vi "_DRIVER_SHARED_INI_VariantToLegibleString.vi"(6 "Format Options":T2, 7 "Preferred Units":T1(array[ring])=[enum."°", enum."m", enum."m²", enum."L", enum."m/s", enum."m/s²", enum."°/s", enum."°/s²", enum."kg", enum."s", enum."Hz", enum."°C", enum."bar", enum."N", enum."kg/m³", enum."N·m", enum."kg·m²", enum."V", enum."A", enum."W", enum."ohm", enum."µF", enum."mH", enum."kW·h", enum."lx", enum."C", enum."eV", enum."Gy", enum."lm", enum."S", enum."T"], 8 "error in (no error)":errorcluster, 11 "Variant":variant) -> (0 "error out":errorcluster, 1 "Var_Value":string, 2 "Var_name":string, 3 "String":string)   [LabVIEW 2020]
doc: "Converts almost anything in the form of a variant into a single line, legible string. Use <b>Format Options</b> to configure the output options. <b>Preferred Units</b> is only used when converting numerics with units. Select the preferred units from the list. If a compatible unit is not found, the base SI units are used."
uses:
  <vilib>/Utility/Data Type/Type Definitions/Data Type.ctl
  <vilib>/Utility/Data Type/NI_Data Type.lvlib
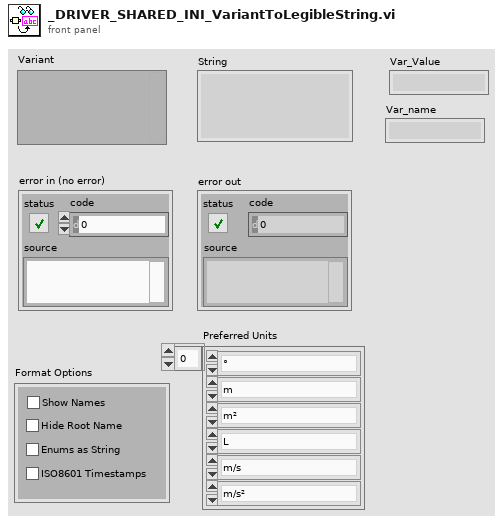
[diagram p1: front panel]
types:
  T1 = enum16{"---- Angle ----", "°", "'", "\"", "rad", "sr", "---- Length ----", "km", "m", "cm", "mm", "µm", "mi", "yd", "ft", "in", "---- Area ----", "ha", "m²", "cm²", "mm²", "µm²", "acre", "yd²", "ft²", "in²", "----Volume ----", "L", "m³", "cm³", "mm³", "gal", "pint", "ft³", "in³", "---- Velocity ----", "km/h", "m/s", "mm/s", "mi/h", "ft/min", "ft/s", "in/s", "---- Accelleration ----", "m/s²", "mm/s²", "ft/s²", "in/s²", "---- Angular Velocity ----", "°/s", "rad/s", "---- Angular Acceleration ----", "°/s²", "rad/s²", "---- Mass ----", "t", "kg", "g", "mg", "µg", "ton", "stone", "lb", "oz", "---- Time ----", "y", "d", "h", "min", "s", "ms", "µs", "ns", "---- Frequency ----", "GHz", "MHz", "kHz", "Hz", "---- Temperature ----", "K", "°C", "°F", "----Pressure ----", "atm", "bar", "mbar", "kPa", "Pa", "mm·Hg", "psi", "---- Force ----", "N", "lbf", "---- Density ----", "g/L", "g/100mL", "mg/L", "kg/m³", "g/cm³", "slug/ft³", "lb/ft³", "---- Torque ----", "N·m", "cN·m", "mN·m", "lb·ft", "oz·in", "---- Inertia ----", "kg·m²", "g·cm²", "lb·ft·s²", "---- Voltage ----", "kV", "V", "mV", "µV", "---- Current ----", "A", "mA", "µA", "---- Power ----", "MW", "kW", "W", "mW", "hp", "---- Resistance ----", "Mohm", "kohm", "ohm", "---- Capacitance ----", "F", "mF", "µF", "nF", "pF", "---- Inductance ----", "H", "mH", "µH", "---- Energy ----", "kW·h", "kJ", "J", "cal", "Btu", "---- Illuminance ----", "lx", "fc", "---- Other ----", "C", "eV", "Gy", "lm", "S", "T"}[]
  T2 = cluster{"Show Names":bool, "Hide Root Name":bool, "Enums as String":bool, "ISO8601 Timestamps":bool}
  T3 = typedef "NI_Data Type.lvlib/Data Type.ctl" = enum8{"Invalid Type", "Void", "I8", "I16", "I32", "I64", "U8", "U16", "U32", "U64", "Single Float", "Double Float", "Extended Float", "Single Complex", "Double Complex", "Extended Complex", "Enum U8", "Enum U16", "Enum U32", "Enum U64", "Single Float With Unit", "Double Float With Unit", "Extended Float With Unit", "Single Complex with Unit", "Double Complex with Unit", "Extended Complex with Unit", "Boolean", "String", "Path", "Picture", "Tag", "Array", "Cluster", "Variant", "LV Variant", "Waveform", "Timestamp", "Digital Waveform", "Digital Data", "ExpressData", "Refnum", "External Data", "VI", "Poly VI", "LabVIEW Class Instance", "Fixed Point", "Set Collection", "Map Collection"}
  T4 = typedef "NI_Data Type.lvlib/Unit Info.ctl" = cluster{"Unit Type":T5, "Exponent":i16}
  T5 = typedef "NI_Data Type.lvlib/Unit Type.ctl" = enum16{"Radians", "Steradians", "Seconds", "Meters", "Kilograms", "Amperes", "Kelvins", "Moles", "Candelas", "InvalidUnit"}
  T6 = typedef "LVFixedPointRepBitsTypeDef.ctl" = cluster{"Signed":bool, "Word Length":u32, "Integer Word Length":i32}
  T7 = typedef "NI_Data Type.lvlib/Refnum Type.ctl" = enum16{"NotARefnum", "UnknownRefnum", "Generic", "Datalog", "ByteStream", "Device", "Occurence", "TCPNetConnection", "Auto", "Menu", "Imaq", "Hardware", "DataSocket", "Visa", "IVI", "UDPNetConnection", "Notifier", "Queue", "Irda", "EventReg", "DotNet", "UserEvent", "Callback", "UNUSED_EMPTY_POSITION", "BlueToothNetConnection", "LVObjApp", "LVObjVI", "LVObjUnknown", "GenericClass", "UserDefinedRefnumTag", "DataValue", "RT FIFO", "TDMS File", "PythonSessionRefnum"}
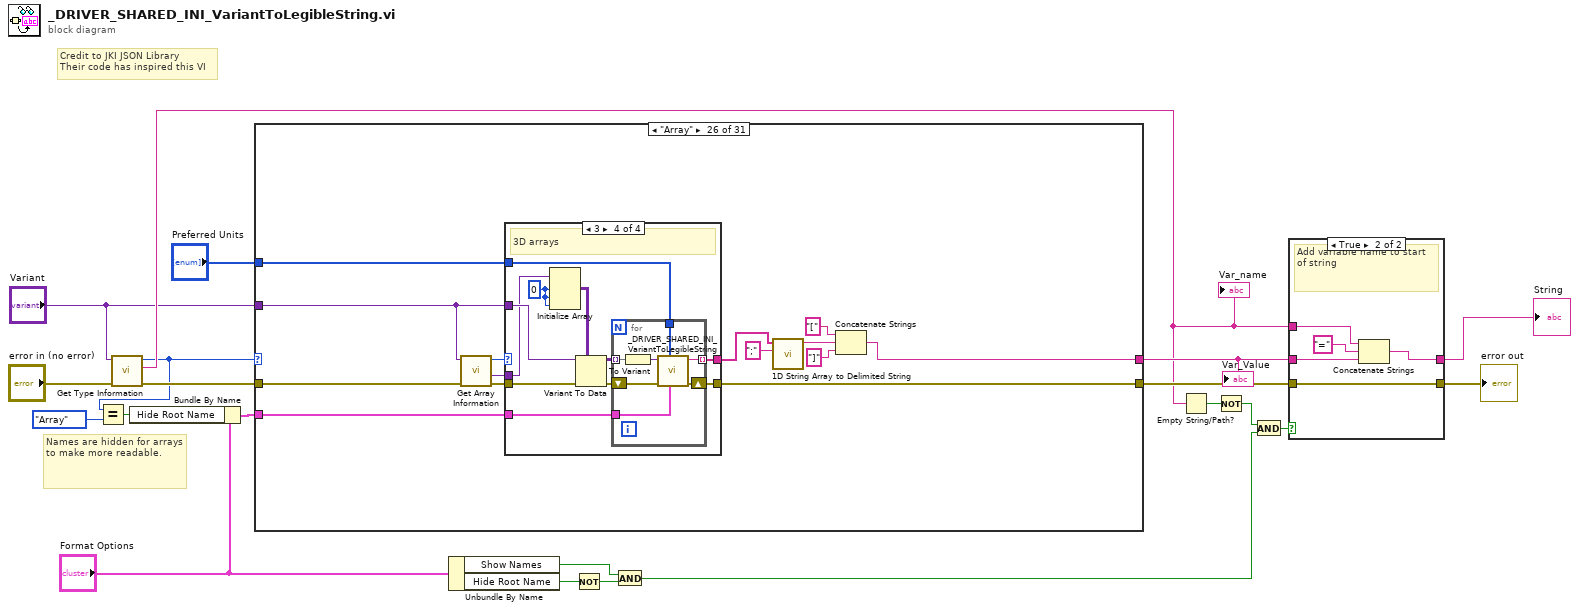
[diagram p0: block diagram]
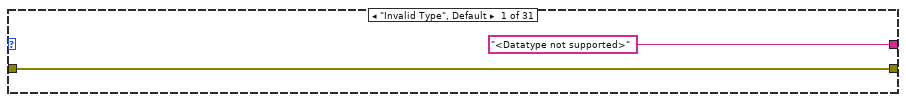
[diagram p3: hidden frame]
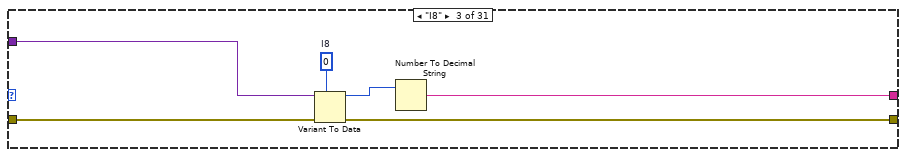
[diagram p5: hidden frame]
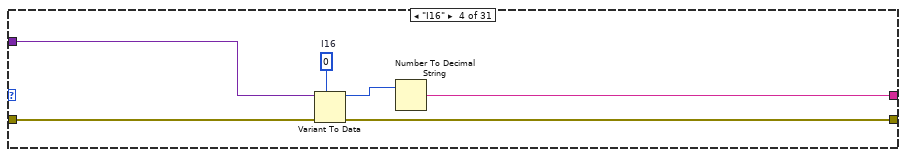
[diagram p6: hidden frame]
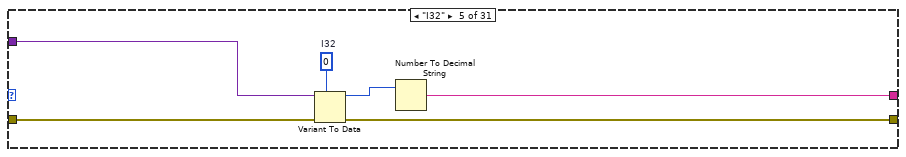
[diagram p7: hidden frame]
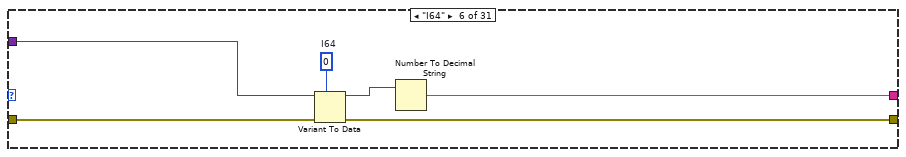
[diagram p8: hidden frame]
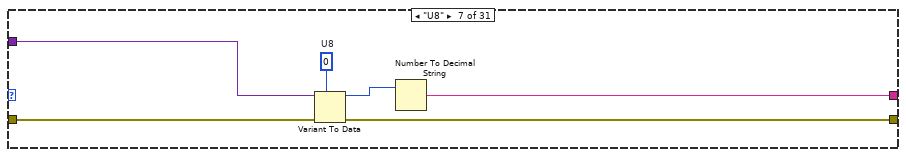
[diagram p9: hidden frame]
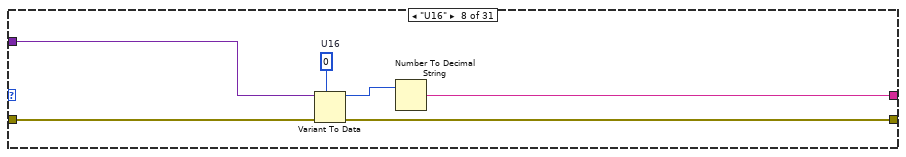
[diagram p10: hidden frame]
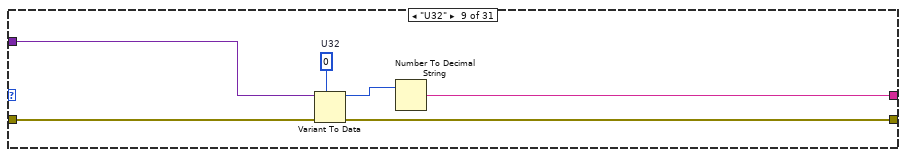
[diagram p11: hidden frame]
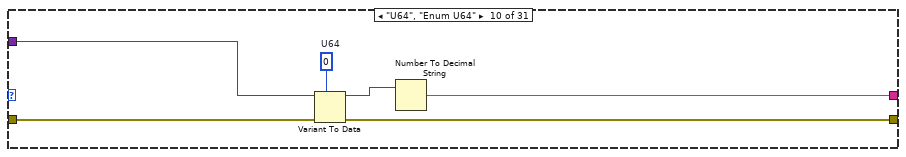
[diagram p12: hidden frame]
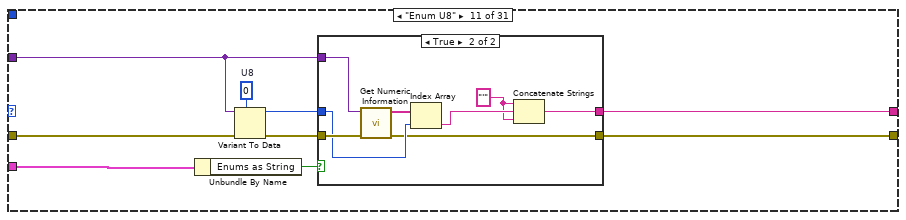
[diagram p13: hidden frame]
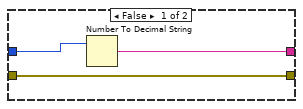
[diagram p14: hidden frame]
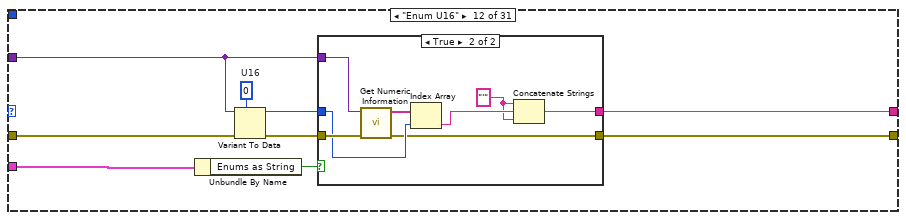
[diagram p15: hidden frame]
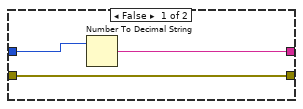
[diagram p16: hidden frame]
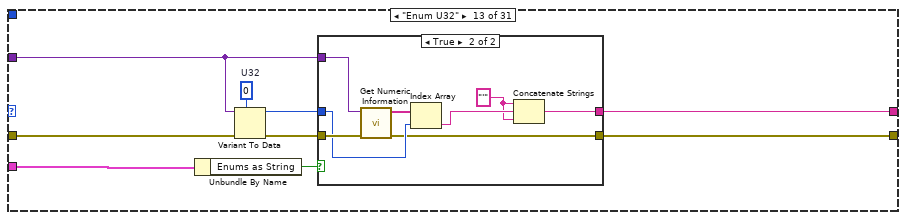
[diagram p17: hidden frame]
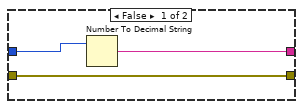
[diagram p18: hidden frame]
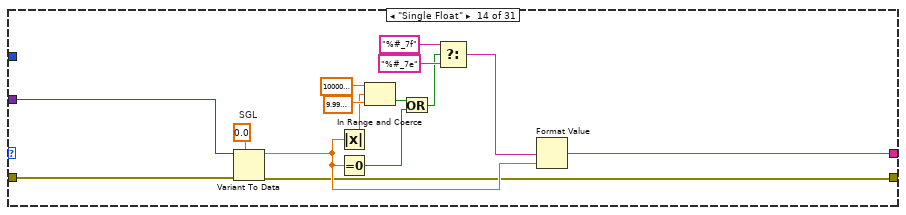
[diagram p19: hidden frame]
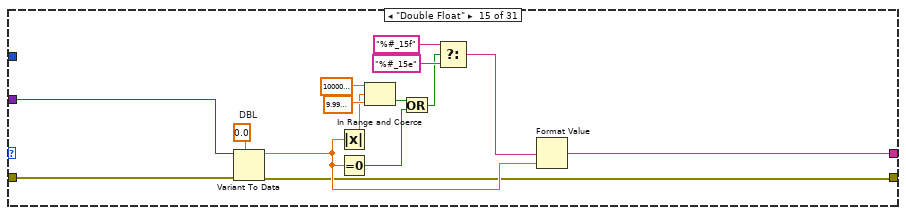
[diagram p20: hidden frame]
diagram:
  # "Names are hidden for arrays  to make more readable."
  # "Credit to JKI JSON Library\nTheir code has inspired this VI"
  n1 = call <vilib>:"Get Type Information.vi"("error in (no error)"="error in (no error)", "variant"="Variant") -> ("error out"=w20:errorcluster, "name"=w15:string, "type"=w5:T3)  [unwired: 5 in, 2 out]
  "Var_name" <- w15
  n2 = Equal?(x=w5, y=Data_Type."Array") -> (x = y?=w3:bool)
  n3 = Bundle By Name(cluster="Format Options", "Hide Root Name"=w3) -> (w6:T2)
  n4 = case shown="\"Array\"" w5 {
    selector: w5 -> [_ _ _ _ _ _ _ _ _ _ _ _ _ _ _ _ w190 _ _ _ _ _ _ _ _ _ _ _ _ _ _]
    tunnel: ["<Datatype not supported>" ("format string") _ w26 w32 w38 w44 w50 w56 w62 w68 w78 w98 w118 w134 w149 w164 w187 w960 w985 w1010 w1046 w1056 w1065 w1074 w1089 w1103 w1173 w1202 w1206 w1235 w1267] -> w16
    tunnel: [w23 w24 w25 w31 w37 w43 w49 w55 w61 w67 w75 w95 w115 w133 w148 w163 w191 w975 w1000 w1025 w1045 w1058 w1064 w1073 w1092 w1112 w1175 w1204 w1207 w1236 w1268] -> w18
    tunnel: w20 -> [w23 w24 w28 w34 w40 w46 w52 w58 w64 w70 w79 w99 w119 w138 w153 w168 w182 w978 w1003 w1028 w1043 w1059 w1069 w1078 w1093 w1113 w1174 w1203 w1213 w1234 w1272]
    tunnel: "Variant" -> [_ _ w27 w33 w39 w45 w51 w57 w63 w69 w76 w96 w116 w137 w152 w167 w180 w977 w1002 w1027 w1041 w1057 w1068 w1077 w1082 w1110 w1172 w1201 w1212 w1231 w1270]
    tunnel: w6 -> [_ _ _ _ _ _ _ _ _ _ w74 w94 w114 _ _ _ _ _ _ _ _ _ _ _ w1086 w1101 w1171 w1191 w1210 _ _]
    tunnel: "Preferred Units" -> [_ _ _ _ _ _ _ _ _ _ _ _ _ _ _ _ w183 _ _ _ _ _ _ _ w1079 w1100 w1170 w1190 _ _ _]
    frame "Invalid Type", Default {
    }
    frame "Void" {
    }
    frame "I8" {
      w29 = i8 0  # I8
      n5 = Variant To Data(error in=w28, type=w29, Variant=w27) -> (data=w30:i8, error out=w25:errorcluster)
      n6 = Number To Decimal String(number=w30) -> (decimal integer string=w26:string)  [unwired: 1 in]
    }
    frame "I16" {
      w35 = i16 0  # I16
      n7 = Variant To Data(error in=w34, type=w35, Variant=w33) -> (data=w36:i16, error out=w31:errorcluster)
      n8 = Number To Decimal String(number=w36) -> (decimal integer string=w32:string)  [unwired: 1 in]
    }
    frame "I32" {
      w41 = 0  # I32
      n9 = Variant To Data(error in=w40, type=w41, Variant=w39) -> (data=w42:i32, error out=w37:errorcluster)
      n10 = Number To Decimal String(number=w42) -> (decimal integer string=w38:string)  [unwired: 1 in]
    }
    frame "I64" {
      w47 = i64 0  # I64
      n11 = Variant To Data(error in=w46, type=w47, Variant=w45) -> (data=w48:i64, error out=w43:errorcluster)
      n12 = Number To Decimal String(number=w48) -> (decimal integer string=w44:string)  [unwired: 1 in]
    }
    frame "U8" {
      w53 = u8 0  # U8
      n13 = Variant To Data(error in=w52, type=w53, Variant=w51) -> (data=w54:u8, error out=w49:errorcluster)
      n14 = Number To Decimal String(number=w54) -> (decimal integer string=w50:string)  [unwired: 1 in]
    }
    frame "U16" {
      w59 = u16 0  # U16
      n15 = Variant To Data(error in=w58, type=w59, Variant=w57) -> (data=w60:u16, error out=w55:errorcluster)
      n16 = Number To Decimal String(number=w60) -> (decimal integer string=w56:string)  [unwired: 1 in]
    }
    frame "U32" {
      w65 = u32 0  # U32
      n17 = Variant To Data(error in=w64, type=w65, Variant=w63) -> (data=w66:u32, error out=w61:errorcluster)
      n18 = Number To Decimal String(number=w66) -> (decimal integer string=w62:string)  [unwired: 1 in]
    }
    frame "U64", "Enum U64" {
      w71 = u64 0  # U64
      n19 = Variant To Data(error in=w70, type=w71, Variant=w69) -> (data=w72:u64, error out=w67:errorcluster)
      n20 = Number To Decimal String(number=w72) -> (decimal integer string=w68:string)  [unwired: 1 in]
    }
    frame "Enum U8" {
      w80 = u8 0  # U8
      n21 = Unbundle By Name(w74) -> ("Enums as String"=w73:bool)
      n22 = Variant To Data(error in=w79, type=w80, Variant=w76) -> (data=w81:u8, error out=w77:errorcluster)
      n23 = case shown="True" w73 {
        tunnel: w81 -> [w84 w89]
        tunnel: [w83 w86] -> w78
        tunnel: w77 -> [w82 w92]
        tunnel: w76 -> [_ w91]
        tunnel: [w82 w88] -> w75
        frame False {
          n24 = Number To Decimal String(number=w84) -> (decimal integer string=w83:string)  [unwired: 1 in]
        }
        frame True {
          w85 = "'" ("string")
          n25 = call <vilib>:"Get Numeric Information.vi"("error in (no error)"=w92, "variant"=w91) -> ("error out"=w88:errorcluster, "enum names"=w90:string[])  [unwired: 6 in, 2 out]
          n26 = Index Array(array=w90, index=w89) -> (element=w87:string)
          n27 = Concatenate Strings(w85, w87, w85) -> (w86:string)
        }
      }
    }
    frame "Enum U16" {
      w100 = u16 0  # U16
      n28 = Unbundle By Name(w94) -> ("Enums as String"=w93:bool)
      n29 = Variant To Data(error in=w99, type=w100, Variant=w96) -> (data=w101:u16, error out=w97:errorcluster)
      n30 = case shown="True" w93 {
        tunnel: w101 -> [w104 w109]
        tunnel: [w103 w106] -> w98
        tunnel: w97 -> [w102 w112]
        tunnel: w96 -> [_ w111]
        tunnel: [w102 w108] -> w95
        frame False {
          n31 = Number To Decimal String(number=w104) -> (decimal integer string=w103:string)  [unwired: 1 in]
        }
        frame True {
          w105 = "'" ("string")
          n32 = call <vilib>:"Get Numeric Information.vi"("error in (no error)"=w112, "variant"=w111) -> ("error out"=w108:errorcluster, "enum names"=w110:string[])  [unwired: 6 in, 2 out]
          n33 = Index Array(array=w110, index=w109) -> (element=w107:string)
          n34 = Concatenate Strings(w105, w107, w105) -> (w106:string)
        }
      }
    }
    frame "Enum U32" {
      w120 = u32 0  # U32
      n35 = Unbundle By Name(w114) -> ("Enums as String"=w113:bool)
      n36 = Variant To Data(error in=w119, type=w120, Variant=w116) -> (data=w121:u32, error out=w117:errorcluster)
      n37 = case shown="True" w113 {
        tunnel: w121 -> [w124 w129]
        tunnel: [w123 w126] -> w118
        tunnel: w117 -> [w122 w132]
        tunnel: w116 -> [_ w131]
        tunnel: [w122 w128] -> w115
        frame False {
          n38 = Number To Decimal String(number=w124) -> (decimal integer string=w123:string)  [unwired: 1 in]
        }
        frame True {
          w125 = "'" ("string")
          n39 = call <vilib>:"Get Numeric Information.vi"("error in (no error)"=w132, "variant"=w131) -> ("error out"=w128:errorcluster, "enum names"=w130:string[])  [unwired: 6 in, 2 out]
          n40 = Index Array(array=w130, index=w129) -> (element=w127:string)
          n41 = Concatenate Strings(w125, w127, w125) -> (w126:string)
        }
      }
    }
    frame "Single Float" {
      w147 = sgl 0.0  # SGL
      n42 = Variant To Data(error in=w138, type=w147, Variant=w137) -> (data=w136:sgl, error out=w133:errorcluster)
      n43 = Absolute Value(x=w136) -> (abs(x)=w143:sgl)
      n44 = Equal To 0?(x=w136) -> (x = 0?=w142:bool)
      n45 = In Range and Coerce(upper limit=1000000.0, x=w143, lower limit=9.999999747378752e-05 ("upper limit")) -> (In Range?=w141:bool)  [unwired: 1 out]
      n46 = Or(x=w141, y=w142) -> (x .or. y?=w140:bool)
      n47 = Select(t="%#_7f" ("format string"), s=w140, f="%#_7e" ("format string")) -> (s? t:f=w135:string)
      n48 = Format Value(format string=w135, value (0)=w136) -> (output string=w134:string)  [unwired: 1 in]
    }
    frame "Double Float" {
      w162 = 0.0  # DBL
      n49 = Variant To Data(error in=w153, type=w162, Variant=w152) -> (data=w151:dbl, error out=w148:errorcluster)
      n50 = Absolute Value(x=w151) -> (abs(x)=w158:dbl)
      n51 = Equal To 0?(x=w151) -> (x = 0?=w157:bool)
      n52 = In Range and Coerce(upper limit=1000000.0, x=w158, lower limit=9.999999747378752e-05 ("upper limit")) -> (In Range?=w156:bool)  [unwired: 1 out]
      n53 = Or(x=w156, y=w157) -> (x .or. y?=w155:bool)
      n54 = Select(t="%#_15f" ("format string"), s=w155, f="%#_15e" ("format string")) -> (s? t:f=w150:string)
      n55 = Format Value(format string=w150, value (0)=w151) -> (output string=w149:string)  [unwired: 1 in]
    }
    frame "Extended Float" {
      w177 = ext 0.0  # EXT
      n56 = Variant To Data(error in=w168, type=w177, Variant=w167) -> (data=w166:ext, error out=w163:errorcluster)
      n57 = Absolute Value(x=w166) -> (abs(x)=w173:ext)
      n58 = Equal To 0?(x=w166) -> (x = 0?=w172:bool)
      n59 = In Range and Coerce(upper limit=1000000.0, x=w173, lower limit=9.999999747378752e-05 ("upper limit")) -> (In Range?=w171:bool)  [unwired: 1 out]
      n60 = Or(x=w171, y=w172) -> (x .or. y?=w170:bool)
      n61 = Select(t="%#_18f" ("format string"), s=w170, f="%#_18e" ("format string")) -> (s? t:f=w165:string)
      n62 = Format Value(format string=w165, value (0)=w166) -> (output string=w164:string)  [unwired: 1 in]
    }
    frame "Single Float With Unit".."Extended Float With Unit" {
      # "Add any new units into this case and update the enum. Copy an existing case and rename with units of choice. The Enum label will become the unit text."
      n63 = for {
        tunnel: w183 -> [w194] mode=indexing
        tunnel: w180 -> [w195]
        tunnel: [w194] -> w181
        tunnel: [w193] -> w179
        tunnel: [w192] -> w178
        stop <- w193 continue-if-true
        # "Search for unit match"
        n64 = case shown="\"mm/s²\"" w194 {
          tunnel: w195 -> [_ w202 w207 w212 w217 w222 w227 w232 w237 w242 w247 w252 w257 w262 w267 w272 w277 w282 w287 w292 w297 w302 w307 w312 w317 w322 w327 w332 w337 w342 w347 w352 w357 w362 w367 w372 w377 w382 w387 w392 w397 w402 w407 w412 w417 w422 w427 w432 w437 w442 w447 w452 w457 w462 w467 w472 w477 w482 w487 w492 w497 w502 w507 w512 w517 w522 w527 w532 w537 w542 w547 w552 w557 w562 w567 w572 w577 w582 w587 w592 w597 w602 w607 w612 w617 w622 w627 w632 w637 w642 w647 w652 w657 w662 w667 w672 w677 w682 w687 w692 w697 w702 w707 w712 w717 w722 w727 w732 w737 w742 w747 w752 w757 w762 w767 w772 w777 w782 w787 w792 w797 w802 w807 w812 w817 w822 w827 w832 w837 w842 w847]
          tunnel: [errorcluster {"status"=TRUE, "code"=0, "source"=""} ("error out") w199 w204 w209 w214 w219 w224 w229 w234 w239 w244 w249 w254 w259 w264 w269 w274 w279 w284 w289 w294 w299 w304 w309 w314 w319 w324 w329 w334 w339 w344 w349 w354 w359 w364 w369 w374 w379 w384 w389 w394 w399 w404 w409 w414 w419 w424 w429 w434 w439 w444 w449 w454 w459 w464 w469 w474 w479 w484 w489 w494 w499 w504 w509 w514 w519 w524 w529 w534 w539 w544 w549 w554 w559 w564 w569 w574 w579 w584 w589 w594 w599 w604 w609 w614 w619 w624 w629 w634 w639 w644 w649 w654 w659 w664 w669 w674 w679 w684 w689 w694 w699 w704 w709 w714 w719 w724 w729 w734 w739 w744 w749 w754 w759 w764 w769 w774 w779 w784 w789 w794 w799 w804 w809 w814 w819 w824 w829 w834 w839 w844] -> w193
          tunnel: [ext 0.0 w198 w203 w208 w213 w218 w223 w228 w233 w238 w243 w248 w253 w258 w263 w268 w273 w278 w283 w288 w293 w298 w303 w308 w313 w318 w323 w328 w333 w338 w343 w348 w353 w358 w363 w368 w373 w378 w383 w388 w393 w398 w403 w408 w413 w418 w423 w428 w433 w438 w443 w448 w453 w458 w463 w468 w473 w478 w483 w488 w493 w498 w503 w508 w513 w518 w523 w528 w533 w538 w543 w548 w553 w558 w563 w568 w573 w578 w583 w588 w593 w598 w603 w608 w613 w618 w623 w628 w633 w638 w643 w648 w653 w658 w663 w668 w673 w678 w683 w688 w693 w698 w703 w708 w713 w718 w723 w728 w733 w738 w743 w748 w753 w758 w763 w768 w773 w778 w783 w788 w793 w798 w803 w808 w813 w818 w823 w828 w833 w838 w843] -> w192
          frame Default {
          }
          frame "°" {
            w201 = ext[unit] 0.0  # deg
            n65 = Variant To Data(type=w201, Variant=w202) -> (data=w200:ext[unit], error out=w199:errorcluster)  [unwired: 1 in]
            n66 = node(w200) -> (w198:ext)
          }
          frame "'" {
            w206 = ext[unit] 0.0  # '
            n67 = Variant To Data(type=w206, Variant=w207) -> (data=w205:ext[unit], error out=w204:errorcluster)  [unwired: 1 in]
            n68 = node(w205) -> (w203:ext)
          }
          frame "\"" {
            w211 = ext[unit] 0.0  # "
            n69 = Variant To Data(type=w211, Variant=w212) -> (data=w210:ext[unit], error out=w209:errorcluster)  [unwired: 1 in]
            n70 = node(w210) -> (w208:ext)
          }
          frame "rad" {
            w216 = ext[unit] 0.0  # rad
            n71 = Variant To Data(type=w216, Variant=w217) -> (data=w215:ext[unit], error out=w214:errorcluster)  [unwired: 1 in]
            n72 = node(w215) -> (w213:ext)
          }
          frame "sr" {
            w221 = ext[unit] 0.0  # sr
            n73 = Variant To Data(type=w221, Variant=w222) -> (data=w220:ext[unit], error out=w219:errorcluster)  [unwired: 1 in]
            n74 = node(w220) -> (w218:ext)
          }
          frame "km" {
            w226 = ext[unit] 0.0  # km
            n75 = Variant To Data(type=w226, Variant=w227) -> (data=w225:ext[unit], error out=w224:errorcluster)  [unwired: 1 in]
            n76 = node(w225) -> (w223:ext)
          }
          frame "m" {
            w231 = ext[unit] 0.0  # m
            n77 = Variant To Data(type=w231, Variant=w232) -> (data=w230:ext[unit], error out=w229:errorcluster)  [unwired: 1 in]
            n78 = node(w230) -> (w228:ext)
          }
          frame "cm" {
            w236 = ext[unit] 0.0  # cm
            n79 = Variant To Data(type=w236, Variant=w237) -> (data=w235:ext[unit], error out=w234:errorcluster)  [unwired: 1 in]
            n80 = node(w235) -> (w233:ext)
          }
          frame "mm" {
            w241 = ext[unit] 0.0  # mm
            n81 = Variant To Data(type=w241, Variant=w242) -> (data=w240:ext[unit], error out=w239:errorcluster)  [unwired: 1 in]
            n82 = node(w240) -> (w238:ext)
          }
          frame "µm" {
            w246 = ext[unit] 0.0  # um
            n83 = Variant To Data(type=w246, Variant=w247) -> (data=w245:ext[unit], error out=w244:errorcluster)  [unwired: 1 in]
            n84 = node(w245) -> (w243:ext)
          }
          frame "mi" {
            w251 = ext[unit] 0.0  # mi
            n85 = Variant To Data(type=w251, Variant=w252) -> (data=w250:ext[unit], error out=w249:errorcluster)  [unwired: 1 in]
            n86 = node(w250) -> (w248:ext)
          }
          frame "yd" {
            w256 = ext[unit] 0.0  # yd
            n87 = Variant To Data(type=w256, Variant=w257) -> (data=w255:ext[unit], error out=w254:errorcluster)  [unwired: 1 in]
            n88 = node(w255) -> (w253:ext)
          }
          frame "ft" {
            w261 = ext[unit] 0.0  # ft
            n89 = Variant To Data(type=w261, Variant=w262) -> (data=w260:ext[unit], error out=w259:errorcluster)  [unwired: 1 in]
            n90 = node(w260) -> (w258:ext)
          }
          frame "in" {
            w266 = ext[unit] 0.0  # in
            n91 = Variant To Data(type=w266, Variant=w267) -> (data=w265:ext[unit], error out=w264:errorcluster)  [unwired: 1 in]
            n92 = node(w265) -> (w263:ext)
          }
          frame "ha" {
            w271 = ext[unit] 0.0  # ha
            n93 = Variant To Data(type=w271, Variant=w272) -> (data=w270:ext[unit], error out=w269:errorcluster)  [unwired: 1 in]
            n94 = node(w270) -> (w268:ext)
          }
          frame "m²" {
            w276 = ext[unit] 0.0  # m^2
            n95 = Variant To Data(type=w276, Variant=w277) -> (data=w275:ext[unit], error out=w274:errorcluster)  [unwired: 1 in]
            n96 = node(w275) -> (w273:ext)
          }
          frame "cm²" {
            w281 = ext[unit] 0.0  # cm^2
            n97 = Variant To Data(type=w281, Variant=w282) -> (data=w280:ext[unit], error out=w279:errorcluster)  [unwired: 1 in]
            n98 = node(w280) -> (w278:ext)
          }
          frame "mm²" {
            w286 = ext[unit] 0.0  # mm^2
            n99 = Variant To Data(type=w286, Variant=w287) -> (data=w285:ext[unit], error out=w284:errorcluster)  [unwired: 1 in]
            n100 = node(w285) -> (w283:ext)
          }
          frame "µm²" {
            w291 = ext[unit] 0.0  # um^2
            n101 = Variant To Data(type=w291, Variant=w292) -> (data=w290:ext[unit], error out=w289:errorcluster)  [unwired: 1 in]
            n102 = node(w290) -> (w288:ext)
          }
          frame "acre" {
            w296 = ext[unit] 0.0  # acre
            n103 = Variant To Data(type=w296, Variant=w297) -> (data=w295:ext[unit], error out=w294:errorcluster)  [unwired: 1 in]
            n104 = node(w295) -> (w293:ext)
          }
          frame "yd²" {
            w301 = ext[unit] 0.0  # yd^2
            n105 = Variant To Data(type=w301, Variant=w302) -> (data=w300:ext[unit], error out=w299:errorcluster)  [unwired: 1 in]
            n106 = node(w300) -> (w298:ext)
          }
          frame "ft²" {
            w306 = ext[unit] 0.0  # ft^2
            n107 = Variant To Data(type=w306, Variant=w307) -> (data=w305:ext[unit], error out=w304:errorcluster)  [unwired: 1 in]
            n108 = node(w305) -> (w303:ext)
          }
          frame "in²" {
            w311 = ext[unit] 0.0  # in^2
            n109 = Variant To Data(type=w311, Variant=w312) -> (data=w310:ext[unit], error out=w309:errorcluster)  [unwired: 1 in]
            n110 = node(w310) -> (w308:ext)
          }
          frame "L" {
            w316 = ext[unit] 0.0  # l
            n111 = Variant To Data(type=w316, Variant=w317) -> (data=w315:ext[unit], error out=w314:errorcluster)  [unwired: 1 in]
            n112 = node(w315) -> (w313:ext)
          }
          frame "m³" {
            w321 = ext[unit] 0.0  # m^3
            n113 = Variant To Data(type=w321, Variant=w322) -> (data=w320:ext[unit], error out=w319:errorcluster)  [unwired: 1 in]
            n114 = node(w320) -> (w318:ext)
          }
          frame "cm³" {
            w326 = ext[unit] 0.0  # cm^3
            n115 = Variant To Data(type=w326, Variant=w327) -> (data=w325:ext[unit], error out=w324:errorcluster)  [unwired: 1 in]
            n116 = node(w325) -> (w323:ext)
          }
          frame "mm³" {
            w331 = ext[unit] 0.0  # mm^3
            n117 = Variant To Data(type=w331, Variant=w332) -> (data=w330:ext[unit], error out=w329:errorcluster)  [unwired: 1 in]
            n118 = node(w330) -> (w328:ext)
          }
          frame "gal" {
            w336 = ext[unit] 0.0  # gal
            n119 = Variant To Data(type=w336, Variant=w337) -> (data=w335:ext[unit], error out=w334:errorcluster)  [unwired: 1 in]
            n120 = node(w335) -> (w333:ext)
          }
          frame "pint" {
            w341 = ext[unit] 0.0  # pint
            n121 = Variant To Data(type=w341, Variant=w342) -> (data=w340:ext[unit], error out=w339:errorcluster)  [unwired: 1 in]
            n122 = node(w340) -> (w338:ext)
          }
          frame "ft³" {
            w346 = ext[unit] 0.0  # ft^3
            n123 = Variant To Data(type=w346, Variant=w347) -> (data=w345:ext[unit], error out=w344:errorcluster)  [unwired: 1 in]
            n124 = node(w345) -> (w343:ext)
          }
          frame "in³" {
            w351 = ext[unit] 0.0  # in^3
            n125 = Variant To Data(type=w351, Variant=w352) -> (data=w350:ext[unit], error out=w349:errorcluster)  [unwired: 1 in]
            n126 = node(w350) -> (w348:ext)
          }
          frame "km/h" {
            w356 = ext[unit] 0.0  # km/h
            n127 = Variant To Data(type=w356, Variant=w357) -> (data=w355:ext[unit], error out=w354:errorcluster)  [unwired: 1 in]
            n128 = node(w355) -> (w353:ext)
          }
          frame "m/s" {
            w361 = ext[unit] 0.0  # m/s
            n129 = Variant To Data(type=w361, Variant=w362) -> (data=w360:ext[unit], error out=w359:errorcluster)  [unwired: 1 in]
            n130 = node(w360) -> (w358:ext)
          }
          frame "mm/s" {
            w366 = ext[unit] 0.0  # mm/s
            n131 = Variant To Data(type=w366, Variant=w367) -> (data=w365:ext[unit], error out=w364:errorcluster)  [unwired: 1 in]
            n132 = node(w365) -> (w363:ext)
          }
          frame "mi/h" {
            w371 = ext[unit] 0.0  # mi/h
            n133 = Variant To Data(type=w371, Variant=w372) -> (data=w370:ext[unit], error out=w369:errorcluster)  [unwired: 1 in]
            n134 = node(w370) -> (w368:ext)
          }
          frame "ft/min" {
            w376 = ext[unit] 0.0  # ft/min
            n135 = Variant To Data(type=w376, Variant=w377) -> (data=w375:ext[unit], error out=w374:errorcluster)  [unwired: 1 in]
            n136 = node(w375) -> (w373:ext)
          }
          frame "ft/s" {
            w381 = ext[unit] 0.0  # ft/s
            n137 = Variant To Data(type=w381, Variant=w382) -> (data=w380:ext[unit], error out=w379:errorcluster)  [unwired: 1 in]
            n138 = node(w380) -> (w378:ext)
          }
          frame "in/s" {
            w386 = ext[unit] 0.0  # in/s
            n139 = Variant To Data(type=w386, Variant=w387) -> (data=w385:ext[unit], error out=w384:errorcluster)  [unwired: 1 in]
            n140 = node(w385) -> (w383:ext)
          }
          frame "m/s²" {
            w391 = ext[unit] 0.0  # m/s^2
            n141 = Variant To Data(type=w391, Variant=w392) -> (data=w390:ext[unit], error out=w389:errorcluster)  [unwired: 1 in]
            n142 = node(w390) -> (w388:ext)
          }
          frame "mm/s²" {
            w396 = ext[unit] 0.0  # mm/s^2
            n143 = Variant To Data(type=w396, Variant=w397) -> (data=w395:ext[unit], error out=w394:errorcluster)  [unwired: 1 in]
            n144 = node(w395) -> (w393:ext)
          }
          frame "ft/s²" {
            w401 = ext[unit] 0.0  # ft/s^2
            n145 = Variant To Data(type=w401, Variant=w402) -> (data=w400:ext[unit], error out=w399:errorcluster)  [unwired: 1 in]
            n146 = node(w400) -> (w398:ext)
          }
          frame "in/s²" {
            w406 = ext[unit] 0.0  # in/s^2
            n147 = Variant To Data(type=w406, Variant=w407) -> (data=w405:ext[unit], error out=w404:errorcluster)  [unwired: 1 in]
            n148 = node(w405) -> (w403:ext)
          }
          frame "°/s" {
            w411 = ext[unit] 0.0  # deg/s
            n149 = Variant To Data(type=w411, Variant=w412) -> (data=w410:ext[unit], error out=w409:errorcluster)  [unwired: 1 in]
            n150 = node(w410) -> (w408:ext)
          }
          frame "rad/s" {
            w416 = ext[unit] 0.0  # rad/s
            n151 = Variant To Data(type=w416, Variant=w417) -> (data=w415:ext[unit], error out=w414:errorcluster)  [unwired: 1 in]
            n152 = node(w415) -> (w413:ext)
          }
          frame "°/s²" {
            w421 = ext[unit] 0.0  # deg/s^2
            n153 = Variant To Data(type=w421, Variant=w422) -> (data=w420:ext[unit], error out=w419:errorcluster)  [unwired: 1 in]
            n154 = node(w420) -> (w418:ext)
          }
          frame "rad/s²" {
            w426 = ext[unit] 0.0  # rad/s^2
            n155 = Variant To Data(type=w426, Variant=w427) -> (data=w425:ext[unit], error out=w424:errorcluster)  [unwired: 1 in]
            n156 = node(w425) -> (w423:ext)
          }
          frame "t" {
            w431 = ext[unit] 0.0  # t
            n157 = Variant To Data(type=w431, Variant=w432) -> (data=w430:ext[unit], error out=w429:errorcluster)  [unwired: 1 in]
            n158 = node(w430) -> (w428:ext)
          }
          frame "kg" {
            w436 = ext[unit] 0.0  # kg
            n159 = Variant To Data(type=w436, Variant=w437) -> (data=w435:ext[unit], error out=w434:errorcluster)  [unwired: 1 in]
            n160 = node(w435) -> (w433:ext)
          }
          frame "g" {
            w441 = ext[unit] 0.0  # g
            n161 = Variant To Data(type=w441, Variant=w442) -> (data=w440:ext[unit], error out=w439:errorcluster)  [unwired: 1 in]
            n162 = node(w440) -> (w438:ext)
          }
          frame "mg" {
            w446 = ext[unit] 0.0  # mg
            n163 = Variant To Data(type=w446, Variant=w447) -> (data=w445:ext[unit], error out=w444:errorcluster)  [unwired: 1 in]
            n164 = node(w445) -> (w443:ext)
          }
          frame "µg" {
            w451 = ext[unit] 0.0  # ug
            n165 = Variant To Data(type=w451, Variant=w452) -> (data=w450:ext[unit], error out=w449:errorcluster)  [unwired: 1 in]
            n166 = node(w450) -> (w448:ext)
          }
          frame "ton" {
            w456 = ext[unit] 0.0  # ton
            n167 = Variant To Data(type=w456, Variant=w457) -> (data=w455:ext[unit], error out=w454:errorcluster)  [unwired: 1 in]
            n168 = node(w455) -> (w453:ext)
          }
          frame "stone" {
            w461 = ext[unit] 0.0  # stone
            n169 = Variant To Data(type=w461, Variant=w462) -> (data=w460:ext[unit], error out=w459:errorcluster)  [unwired: 1 in]
            n170 = node(w460) -> (w458:ext)
          }
          frame "lb" {
            w466 = ext[unit] 0.0  # lb
            n171 = Variant To Data(type=w466, Variant=w467) -> (data=w465:ext[unit], error out=w464:errorcluster)  [unwired: 1 in]
            n172 = node(w465) -> (w463:ext)
          }
          frame "oz" {
            w471 = ext[unit] 0.0  # oz
            n173 = Variant To Data(type=w471, Variant=w472) -> (data=w470:ext[unit], error out=w469:errorcluster)  [unwired: 1 in]
            n174 = node(w470) -> (w468:ext)
          }
          frame "y" {
            w476 = ext[unit] 0.0  # a
            n175 = Variant To Data(type=w476, Variant=w477) -> (data=w475:ext[unit], error out=w474:errorcluster)  [unwired: 1 in]
            n176 = node(w475) -> (w473:ext)
          }
          frame "d" {
            w481 = ext[unit] 0.0  # d
            n177 = Variant To Data(type=w481, Variant=w482) -> (data=w480:ext[unit], error out=w479:errorcluster)  [unwired: 1 in]
            n178 = node(w480) -> (w478:ext)
          }
          frame "h" {
            w486 = ext[unit] 0.0  # h
            n179 = Variant To Data(type=w486, Variant=w487) -> (data=w485:ext[unit], error out=w484:errorcluster)  [unwired: 1 in]
            n180 = node(w485) -> (w483:ext)
          }
          frame "min" {
            w491 = ext[unit] 0.0  # min
            n181 = Variant To Data(type=w491, Variant=w492) -> (data=w490:ext[unit], error out=w489:errorcluster)  [unwired: 1 in]
            n182 = node(w490) -> (w488:ext)
          }
          frame "s" {
            w496 = ext[unit] 0.0  # s
            n183 = Variant To Data(type=w496, Variant=w497) -> (data=w495:ext[unit], error out=w494:errorcluster)  [unwired: 1 in]
            n184 = node(w495) -> (w493:ext)
          }
          frame "ms" {
            w501 = ext[unit] 0.0  # ms
            n185 = Variant To Data(type=w501, Variant=w502) -> (data=w500:ext[unit], error out=w499:errorcluster)  [unwired: 1 in]
            n186 = node(w500) -> (w498:ext)
          }
          frame "µs" {
            w506 = ext[unit] 0.0  # us
            n187 = Variant To Data(type=w506, Variant=w507) -> (data=w505:ext[unit], error out=w504:errorcluster)  [unwired: 1 in]
            n188 = node(w505) -> (w503:ext)
          }
          frame "ns" {
            w511 = ext[unit] 0.0  # ns
            n189 = Variant To Data(type=w511, Variant=w512) -> (data=w510:ext[unit], error out=w509:errorcluster)  [unwired: 1 in]
            n190 = node(w510) -> (w508:ext)
          }
          frame "GHz" {
            w516 = ext[unit] 0.0  # GHz
            n191 = Variant To Data(type=w516, Variant=w517) -> (data=w515:ext[unit], error out=w514:errorcluster)  [unwired: 1 in]
            n192 = node(w515) -> (w513:ext)
          }
          frame "MHz" {
            w521 = ext[unit] 0.0  # MHz
            n193 = Variant To Data(type=w521, Variant=w522) -> (data=w520:ext[unit], error out=w519:errorcluster)  [unwired: 1 in]
            n194 = node(w520) -> (w518:ext)
          }
          frame "kHz" {
            w526 = ext[unit] 0.0  # kHz
            n195 = Variant To Data(type=w526, Variant=w527) -> (data=w525:ext[unit], error out=w524:errorcluster)  [unwired: 1 in]
            n196 = node(w525) -> (w523:ext)
          }
          frame "Hz" {
            w531 = ext[unit] 0.0  # Hz
            n197 = Variant To Data(type=w531, Variant=w532) -> (data=w530:ext[unit], error out=w529:errorcluster)  [unwired: 1 in]
            n198 = node(w530) -> (w528:ext)
          }
          frame "K" {
            w536 = ext[unit] 0.0  # K
            n199 = Variant To Data(type=w536, Variant=w537) -> (data=w535:ext[unit], error out=w534:errorcluster)  [unwired: 1 in]
            n200 = node(w535) -> (w533:ext)
          }
          frame "°C" {
            w541 = ext[unit] 273.15  # degC
            n201 = Variant To Data(type=w541, Variant=w542) -> (data=w540:ext[unit], error out=w539:errorcluster)  [unwired: 1 in]
            n202 = node(w540) -> (w538:ext)
          }
          frame "°F" {
            w546 = ext[unit] 255.3722222222222  # degF
            n203 = Variant To Data(type=w546, Variant=w547) -> (data=w545:ext[unit], error out=w544:errorcluster)  [unwired: 1 in]
            n204 = node(w545) -> (w543:ext)
          }
          frame "atm" {
            w551 = ext[unit] 0.0  # atm
            n205 = Variant To Data(type=w551, Variant=w552) -> (data=w550:ext[unit], error out=w549:errorcluster)  [unwired: 1 in]
            n206 = node(w550) -> (w548:ext)
          }
          frame "bar" {
            w556 = ext[unit] 0.0  # bar
            n207 = Variant To Data(type=w556, Variant=w557) -> (data=w555:ext[unit], error out=w554:errorcluster)  [unwired: 1 in]
            n208 = node(w555) -> (w553:ext)
          }
          frame "mbar" {
            w561 = ext[unit] 0.0  # mbar
            n209 = Variant To Data(type=w561, Variant=w562) -> (data=w560:ext[unit], error out=w559:errorcluster)  [unwired: 1 in]
            n210 = node(w560) -> (w558:ext)
          }
          frame "kPa" {
            w566 = ext[unit] 0.0  # kPa
            n211 = Variant To Data(type=w566, Variant=w567) -> (data=w565:ext[unit], error out=w564:errorcluster)  [unwired: 1 in]
            n212 = node(w565) -> (w563:ext)
          }
          frame "Pa" {
            w571 = ext[unit] 0.0  # Pa
            n213 = Variant To Data(type=w571, Variant=w572) -> (data=w570:ext[unit], error out=w569:errorcluster)  [unwired: 1 in]
            n214 = node(w570) -> (w568:ext)
          }
          frame "mm·Hg" {
            w576 = ext[unit] 0.0  # mm.Hg
            n215 = Variant To Data(type=w576, Variant=w577) -> (data=w575:ext[unit], error out=w574:errorcluster)  [unwired: 1 in]
            n216 = node(w575) -> (w573:ext)
          }
          frame "psi" {
            w581 = ext[unit] 0.0  # psi
            n217 = Variant To Data(type=w581, Variant=w582) -> (data=w580:ext[unit], error out=w579:errorcluster)  [unwired: 1 in]
            n218 = node(w580) -> (w578:ext)
          }
          frame "N" {
            w586 = ext[unit] 0.0  # N
            n219 = Variant To Data(type=w586, Variant=w587) -> (data=w585:ext[unit], error out=w584:errorcluster)  [unwired: 1 in]
            n220 = node(w585) -> (w583:ext)
          }
          frame "lbf" {
            w591 = ext[unit] 0.0  # lbf
            n221 = Variant To Data(type=w591, Variant=w592) -> (data=w590:ext[unit], error out=w589:errorcluster)  [unwired: 1 in]
            n222 = node(w590) -> (w588:ext)
          }
          frame "g/L" {
            w596 = ext[unit] 0.0  # g/l
            n223 = Variant To Data(type=w596, Variant=w597) -> (data=w595:ext[unit], error out=w594:errorcluster)  [unwired: 1 in]
            n224 = node(w595) -> (w593:ext)
          }
          frame "mg/L" {
            w601 = ext[unit] 0.0  # mg/l
            n225 = Variant To Data(type=w601, Variant=w602) -> (data=w600:ext[unit], error out=w599:errorcluster)  [unwired: 1 in]
            n226 = node(w600) -> (w598:ext)
          }
          frame "g/100mL" {
            w606 = ext[unit] 0.0  # g/dl
            n227 = Variant To Data(type=w606, Variant=w607) -> (data=w605:ext[unit], error out=w604:errorcluster)  [unwired: 1 in]
            n228 = node(w605) -> (w603:ext)
          }
          frame "kg/m³" {
            w611 = ext[unit] 0.0  # kg/m^3
            n229 = Variant To Data(type=w611, Variant=w612) -> (data=w610:ext[unit], error out=w609:errorcluster)  [unwired: 1 in]
            n230 = node(w610) -> (w608:ext)
          }
          frame "g/cm³" {
            w616 = ext[unit] 0.0  # g/cm^3
            n231 = Variant To Data(type=w616, Variant=w617) -> (data=w615:ext[unit], error out=w614:errorcluster)  [unwired: 1 in]
            n232 = node(w615) -> (w613:ext)
          }
          frame "slug/ft³" {
            w621 = ext[unit] 0.0  # slug/ft^3
            n233 = Variant To Data(type=w621, Variant=w622) -> (data=w620:ext[unit], error out=w619:errorcluster)  [unwired: 1 in]
            n234 = node(w620) -> (w618:ext)
          }
          frame "lb/ft³" {
            w626 = ext[unit] 0.0  # lb/ft^3
            n235 = Variant To Data(type=w626, Variant=w627) -> (data=w625:ext[unit], error out=w624:errorcluster)  [unwired: 1 in]
            n236 = node(w625) -> (w623:ext)
          }
          frame "N·m" {
            w631 = ext[unit] 0.0  # N m
            n237 = Variant To Data(type=w631, Variant=w632) -> (data=w630:ext[unit], error out=w629:errorcluster)  [unwired: 1 in]
            n238 = node(w630) -> (w628:ext)
          }
          frame "cN·m" {
            w636 = ext[unit] 0.0  # cN m
            n239 = Variant To Data(type=w636, Variant=w637) -> (data=w635:ext[unit], error out=w634:errorcluster)  [unwired: 1 in]
            n240 = node(w635) -> (w633:ext)
          }
          frame "mN·m" {
            w641 = ext[unit] 0.0  # mN m
            n241 = Variant To Data(type=w641, Variant=w642) -> (data=w640:ext[unit], error out=w639:errorcluster)  [unwired: 1 in]
            n242 = node(w640) -> (w638:ext)
          }
          frame "lb·ft" {
            w646 = ext[unit] 0.0  # lb ft
            n243 = Variant To Data(type=w646, Variant=w647) -> (data=w645:ext[unit], error out=w644:errorcluster)  [unwired: 1 in]
            n244 = node(w645) -> (w643:ext)
          }
          frame "oz·in" {
            w651 = ext[unit] 0.0  # oz in
            n245 = Variant To Data(type=w651, Variant=w652) -> (data=w650:ext[unit], error out=w649:errorcluster)  [unwired: 1 in]
            n246 = node(w650) -> (w648:ext)
          }
          frame "kg·m²" {
            w656 = ext[unit] 0.0  # kg m^2
            n247 = Variant To Data(type=w656, Variant=w657) -> (data=w655:ext[unit], error out=w654:errorcluster)  [unwired: 1 in]
            n248 = node(w655) -> (w653:ext)
          }
          frame "g·cm²" {
            w661 = ext[unit] 0.0  # g cm^2
            n249 = Variant To Data(type=w661, Variant=w662) -> (data=w660:ext[unit], error out=w659:errorcluster)  [unwired: 1 in]
            n250 = node(w660) -> (w658:ext)
          }
          frame "lb·ft·s²" {
            w666 = ext[unit] 0.0  # lb ft s^2
            n251 = Variant To Data(type=w666, Variant=w667) -> (data=w665:ext[unit], error out=w664:errorcluster)  [unwired: 1 in]
            n252 = node(w665) -> (w663:ext)
          }
          frame "kV" {
            w671 = ext[unit] 0.0  # kV
            n253 = Variant To Data(type=w671, Variant=w672) -> (data=w670:ext[unit], error out=w669:errorcluster)  [unwired: 1 in]
            n254 = node(w670) -> (w668:ext)
          }
          frame "V" {
            w676 = ext[unit] 0.0  # V
            n255 = Variant To Data(type=w676, Variant=w677) -> (data=w675:ext[unit], error out=w674:errorcluster)  [unwired: 1 in]
            n256 = node(w675) -> (w673:ext)
          }
          frame "mV" {
            w681 = ext[unit] 0.0  # mV
            n257 = Variant To Data(type=w681, Variant=w682) -> (data=w680:ext[unit], error out=w679:errorcluster)  [unwired: 1 in]
            n258 = node(w680) -> (w678:ext)
          }
          frame "µV" {
            w686 = ext[unit] 0.0  # uV
            n259 = Variant To Data(type=w686, Variant=w687) -> (data=w685:ext[unit], error out=w684:errorcluster)  [unwired: 1 in]
            n260 = node(w685) -> (w683:ext)
          }
          frame "A" {
            w691 = ext[unit] 0.0  # A
            n261 = Variant To Data(type=w691, Variant=w692) -> (data=w690:ext[unit], error out=w689:errorcluster)  [unwired: 1 in]
            n262 = node(w690) -> (w688:ext)
          }
          frame "mA" {
            w696 = ext[unit] 0.0  # mA
            n263 = Variant To Data(type=w696, Variant=w697) -> (data=w695:ext[unit], error out=w694:errorcluster)  [unwired: 1 in]
            n264 = node(w695) -> (w693:ext)
          }
          frame "µA" {
            w701 = ext[unit] 0.0  # uA
            n265 = Variant To Data(type=w701, Variant=w702) -> (data=w700:ext[unit], error out=w699:errorcluster)  [unwired: 1 in]
            n266 = node(w700) -> (w698:ext)
          }
          frame "MW" {
            w706 = ext[unit] 0.0  # MW
            n267 = Variant To Data(type=w706, Variant=w707) -> (data=w705:ext[unit], error out=w704:errorcluster)  [unwired: 1 in]
            n268 = node(w705) -> (w703:ext)
          }
          frame "kW" {
            w711 = ext[unit] 0.0  # kW
            n269 = Variant To Data(type=w711, Variant=w712) -> (data=w710:ext[unit], error out=w709:errorcluster)  [unwired: 1 in]
            n270 = node(w710) -> (w708:ext)
          }
          frame "W" {
            w716 = ext[unit] 0.0  # W
            n271 = Variant To Data(type=w716, Variant=w717) -> (data=w715:ext[unit], error out=w714:errorcluster)  [unwired: 1 in]
            n272 = node(w715) -> (w713:ext)
          }
          frame "mW" {
            w721 = ext[unit] 0.0  # mW
            n273 = Variant To Data(type=w721, Variant=w722) -> (data=w720:ext[unit], error out=w719:errorcluster)  [unwired: 1 in]
            n274 = node(w720) -> (w718:ext)
          }
          frame "hp" {
            w726 = ext[unit] 0.0  # hp
            n275 = Variant To Data(type=w726, Variant=w727) -> (data=w725:ext[unit], error out=w724:errorcluster)  [unwired: 1 in]
            n276 = node(w725) -> (w723:ext)
          }
          frame "Mohm" {
            w731 = ext[unit] 0.0  # MOhm
            n277 = Variant To Data(type=w731, Variant=w732) -> (data=w730:ext[unit], error out=w729:errorcluster)  [unwired: 1 in]
            n278 = node(w730) -> (w728:ext)
          }
          frame "kohm" {
            w736 = ext[unit] 0.0  # kOhm
            n279 = Variant To Data(type=w736, Variant=w737) -> (data=w735:ext[unit], error out=w734:errorcluster)  [unwired: 1 in]
            n280 = node(w735) -> (w733:ext)
          }
          frame "ohm" {
            w741 = ext[unit] 0.0  # Ohm
            n281 = Variant To Data(type=w741, Variant=w742) -> (data=w740:ext[unit], error out=w739:errorcluster)  [unwired: 1 in]
            n282 = node(w740) -> (w738:ext)
          }
          frame "F" {
            w746 = ext[unit] 0.0  # F
            n283 = Variant To Data(type=w746, Variant=w747) -> (data=w745:ext[unit], error out=w744:errorcluster)  [unwired: 1 in]
            n284 = node(w745) -> (w743:ext)
          }
          frame "mF" {
            w751 = ext[unit] 0.0  # mF
            n285 = Variant To Data(type=w751, Variant=w752) -> (data=w750:ext[unit], error out=w749:errorcluster)  [unwired: 1 in]
            n286 = node(w750) -> (w748:ext)
          }
          frame "µF" {
            w756 = ext[unit] 0.0  # uF
            n287 = Variant To Data(type=w756, Variant=w757) -> (data=w755:ext[unit], error out=w754:errorcluster)  [unwired: 1 in]
            n288 = node(w755) -> (w753:ext)
          }
          frame "nF" {
            w761 = ext[unit] 0.0  # nF
            n289 = Variant To Data(type=w761, Variant=w762) -> (data=w760:ext[unit], error out=w759:errorcluster)  [unwired: 1 in]
            n290 = node(w760) -> (w758:ext)
          }
          frame "pF" {
            w766 = ext[unit] 0.0  # pF
            n291 = Variant To Data(type=w766, Variant=w767) -> (data=w765:ext[unit], error out=w764:errorcluster)  [unwired: 1 in]
            n292 = node(w765) -> (w763:ext)
          }
          frame "H" {
            w771 = ext[unit] 0.0  # H
            n293 = Variant To Data(type=w771, Variant=w772) -> (data=w770:ext[unit], error out=w769:errorcluster)  [unwired: 1 in]
            n294 = node(w770) -> (w768:ext)
          }
          frame "mH" {
            w776 = ext[unit] 0.0  # mH
            n295 = Variant To Data(type=w776, Variant=w777) -> (data=w775:ext[unit], error out=w774:errorcluster)  [unwired: 1 in]
            n296 = node(w775) -> (w773:ext)
          }
          frame "µH" {
            w781 = ext[unit] 0.0  # uH
            n297 = Variant To Data(type=w781, Variant=w782) -> (data=w780:ext[unit], error out=w779:errorcluster)  [unwired: 1 in]
            n298 = node(w780) -> (w778:ext)
          }
          frame "kW·h" {
            w786 = ext[unit] 0.0  # kW h
            n299 = Variant To Data(type=w786, Variant=w787) -> (data=w785:ext[unit], error out=w784:errorcluster)  [unwired: 1 in]
            n300 = node(w785) -> (w783:ext)
          }
          frame "kJ" {
            w791 = ext[unit] 0.0  # kJ
            n301 = Variant To Data(type=w791, Variant=w792) -> (data=w790:ext[unit], error out=w789:errorcluster)  [unwired: 1 in]
            n302 = node(w790) -> (w788:ext)
          }
          frame "J" {
            w796 = ext[unit] 0.0  # J
            n303 = Variant To Data(type=w796, Variant=w797) -> (data=w795:ext[unit], error out=w794:errorcluster)  [unwired: 1 in]
            n304 = node(w795) -> (w793:ext)
          }
          frame "cal" {
            w801 = ext[unit] 0.0  # cal
            n305 = Variant To Data(type=w801, Variant=w802) -> (data=w800:ext[unit], error out=w799:errorcluster)  [unwired: 1 in]
            n306 = node(w800) -> (w798:ext)
          }
          frame "Btu" {
            w806 = ext[unit] 0.0  # Btu
            n307 = Variant To Data(type=w806, Variant=w807) -> (data=w805:ext[unit], error out=w804:errorcluster)  [unwired: 1 in]
            n308 = node(w805) -> (w803:ext)
          }
          frame "lx" {
            w811 = ext[unit] 0.0  # lx
            n309 = Variant To Data(type=w811, Variant=w812) -> (data=w810:ext[unit], error out=w809:errorcluster)  [unwired: 1 in]
            n310 = node(w810) -> (w808:ext)
          }
          frame "fc" {
            w816 = ext[unit] 0.0  # fc
            n311 = Variant To Data(type=w816, Variant=w817) -> (data=w815:ext[unit], error out=w814:errorcluster)  [unwired: 1 in]
            n312 = node(w815) -> (w813:ext)
          }
          frame "C" {
            w821 = ext[unit] 0.0  # C
            n313 = Variant To Data(type=w821, Variant=w822) -> (data=w820:ext[unit], error out=w819:errorcluster)  [unwired: 1 in]
            n314 = node(w820) -> (w818:ext)
          }
          frame "eV" {
            w826 = ext[unit] 0.0  # eV
            n315 = Variant To Data(type=w826, Variant=w827) -> (data=w825:ext[unit], error out=w824:errorcluster)  [unwired: 1 in]
            n316 = node(w825) -> (w823:ext)
          }
          frame "Gy" {
            w831 = ext[unit] 0.0  # Gy
            n317 = Variant To Data(type=w831, Variant=w832) -> (data=w830:ext[unit], error out=w829:errorcluster)  [unwired: 1 in]
            n318 = node(w830) -> (w828:ext)
          }
          frame "lm" {
            w836 = ext[unit] 0.0  # lm
            n319 = Variant To Data(type=w836, Variant=w837) -> (data=w835:ext[unit], error out=w834:errorcluster)  [unwired: 1 in]
            n320 = node(w835) -> (w833:ext)
          }
          frame "S" {
            w841 = ext[unit] 0.0  # S
            n321 = Variant To Data(type=w841, Variant=w842) -> (data=w840:ext[unit], error out=w839:errorcluster)  [unwired: 1 in]
            n322 = node(w840) -> (w838:ext)
          }
          frame "T" {
            w846 = ext[unit] 0.0  # T
            n323 = Variant To Data(type=w846, Variant=w847) -> (data=w845:ext[unit], error out=w844:errorcluster)  [unwired: 1 in]
            n324 = node(w845) -> (w843:ext)
          }
        }
      }
      n325 = case shown="\"Double Float With Unit\"" w190 {
        tunnel: ["%#_7e" ("format string") "%#_15e" ("format string") "%#_18e" ("format string")] -> w185
        tunnel: ["%#_7f" ("format string") "%#_15f" ("format string") "%#_18f" ("format string")] -> w186
        frame "Single Float With Unit", Default {
        }
        frame "Double Float With Unit" {
        }
        frame "Extended Float With Unit" {
        }
      }
      n326 = case shown="Error" w179 {
        tunnel: [w867 w895] -> w188
        tunnel: w181 -> [w868 _]
        tunnel: w180 -> [_ w872]
        tunnel: [w855 w874] -> w191
        tunnel: w182 -> [w866 w875]
        tunnel: w178 -> [w854 _]
        tunnel: w186 -> [w856 w880]
        tunnel: w185 -> [w857 w879]
        tunnel: [w858 w878] -> w184
        frame No Error {
          # "Match with preferred unit found. Get unit string from enum and format value."
          n327 = To Variant(anything=w868) -> (Variant=w869:variant)
          n328 = call <vilib>:"Get Numeric Information.vi"("error in (no error)"=w866, "variant"=w869) -> ("error out"=w855:errorcluster, "enum names"=w870:string[])  [unwired: 6 in, 2 out]
          n329 = Index Array(array=w870, index=w868) -> (element=w867:string)
          n330 = Absolute Value(x=w854) -> (abs(x)=w865:ext)
          n331 = Equal To 0?(x=w854) -> (x = 0?=w864:bool)
          n332 = In Range and Coerce(upper limit=ext 1000000.0, x=w865, lower limit=ext 9.999999747378752e-05 ("upper limit")) -> (In Range?=w863:bool)  [unwired: 1 out]
          n333 = Or(x=w863, y=w864) -> (x .or. y?=w862:bool)
          n334 = Select(t=w856, s=w862, f=w857) -> (s? t:f=w861:string)
          n335 = Format Value(format string=w861, value (0)=w854) -> (output string=w858:string)  [unwired: 1 in]
        }
        frame Error {
          w876 = ext 0.0  # EXT
          w894 = "·"
          # "denominator"
          # "numerator"
          # "Sort by exponent"
          # "No match found. Construct unit string with SI base units."
          n336 = call <vilib>:"Get Numeric Information.vi"("error in (no error)"=w875, "variant"=w872) -> ("error out"=w877:errorcluster, "units"=w873:T4[])  [unwired: 6 in, 2 out]
          n337 = for {
            tunnel: w873 -> [w904] mode=indexing
            tunnel: [w901] -> w891 mode=indexing
            n338 = Unbundle(w904) -> ("Unit Type"=w902:T5, "Exponent"=w903:i16)
            n339 = Bundle("Exponent"=w903, "Unit Type"=w902) -> (w901:cluster{"Exponent":i16, "Unit Type":T5})  [unwired: 1 in]
          }
          n340 = Variant To Data(error in=w877, type=w876, Variant=w872) -> (data=w871:ext, error out=w874:errorcluster)
          n341 = Sort 1D Array(array=w891) -> (sorted array=w890:cluster{"Exponent":i16, "Unit Type":T5}[])
          n342 = for {
            tunnel: w890 -> [w935] mode=indexing
            tunnel: [w930] -> w900 mode=indexing if=w928
            tunnel: [w930] -> w889 mode=indexing if=w929
            n343 = Unbundle By Name(w935) -> ("Unit Type"=w934:T5, "Exponent"=w933:i16)
            n344 = case shown="\"InvalidUnit\", Default" w934 {
              tunnel: ["rad" "s" "m" "kg" "A" "sr" "K" "mol" "cd" ""] -> w931
              frame "Radians" {
              }
              frame "Seconds" {
              }
              frame "Meters" {
              }
              frame "Kilograms" {
              }
              frame "Amperes" {
              }
              frame "Steradians" {
              }
              frame "Kelvins" {
              }
              frame "Moles" {
              }
              frame "Candelas" {
              }
              frame "InvalidUnit", Default {
              }
            }
            n345 = Absolute Value(x=w933) -> (abs(x)=w932:i16)
            n346 = Greater Than 0?(x=w933) -> (x > 0?=w928:bool)
            n347 = case shown="Default" w932 {
              selector: w932 -> [_ _ _ _ w948]
              tunnel: w931 -> [_ w937 w940 w943 w947]
              tunnel: ["" w937 w938 w941 w944] -> w930
              frame 0 {
              }
              frame 1 {
              }
              frame 2 {
                n348 = Concatenate Strings(w940, "²" ("string")) -> (w938:string)
              }
              frame 3 {
                n349 = Concatenate Strings(w943, "³" ("string")) -> (w941:string)
              }
              frame Default {
                n350 = Number To Decimal String(number=w948) -> (decimal integer string=w946:string)  [unwired: 1 in]
                n351 = Concatenate Strings(w947, "^" ("string"), w946) -> (w944:string)
              }
            }
            n352 = Not(x=w928) -> (.not. x?=w929:bool)
          }
          n353 = Absolute Value(x=w871) -> (abs(x)=w887:ext)
          n354 = Equal To 0?(x=w871) -> (x = 0?=w886:bool)
          n355 = In Range and Coerce(upper limit=ext 1000000.0, x=w887, lower limit=ext 9.999999747378752e-05 ("upper limit")) -> (In Range?=w885:bool)  [unwired: 1 out]
          n356 = call <vilib>:"1D String Array to Delimited String.vi"("delimiter"=w894, "string array"=w900) -> ("delimited string"=w899:string)  [unwired: 9 in]
          n357 = Array Size(array=w900) -> (size(s)=w898:i32)
          n358 = Array Size(array=w889) -> (size(s)=w893:i32)
          n359 = Reverse 1D Array(array=w889) -> (reversed array=w888:string[])
          n360 = Or(x=w885, y=w886) -> (x .or. y?=w884:bool)
          n361 = Equal To 0?(x=w893) -> (x = 0?=w892:bool)
          n362 = call <vilib>:"1D String Array to Delimited String.vi"("delimiter"=w894, "string array"=w888) -> ("delimited string"=w897:string)  [unwired: 9 in]
          n363 = case shown="Default" w898 {
            tunnel: w899 -> [w915 _ w922]
            tunnel: [w915 w917 w921] -> w896
            tunnel: w892 -> [_ w916 w920]
            frame 1 {
            }
            frame 0 {
              n364 = case shown="True" w916 {
                tunnel: ["1" ("delimited string") ""] -> w917
                frame False {
                }
                frame True {
                }
              }
            }
            frame Default {
              n365 = case shown="False" w920 {
                tunnel: w922 -> [w926 w927]
                tunnel: [w923 w927] -> w921
                frame False {
                  n366 = Concatenate Strings("(" ("string"), w926, ")" ("string")) -> (w923:string)
                }
                frame True {
                }
              }
            }
          }
          n367 = Select(t=w880, s=w884, f=w879) -> (s? t:f=w883:string)
          n368 = case shown="Default" w893 {
            tunnel: w897 -> [w906 _ w914]
            tunnel: [w907 w909 w912] -> w895
            tunnel: w896 -> [w908 w909 w910]
            frame 1 {
              n369 = Concatenate Strings(w908, "/" ("string"), w906) -> (w907:string)
            }
            frame 0 {
            }
            frame Default {
              n370 = Concatenate Strings(w910, "/(" ("string"), w914, ")" ("string")) -> (w912:string)
            }
          }
          n371 = Format Value(format string=w883, value (0)=w871) -> (output string=w878:string)  [unwired: 1 in]
        }
      }
      n372 = call <vilib>:"Space Constant.vi"() -> ("String"=w189:string)
      n373 = Concatenate Strings(w184, w189, w188) -> (w187:string)
    }
    frame "Single Complex" {
      w967 = "%#_7e" ("format string")
      w966 = "%#_7f" ("format string")
      w983 = csg 0.0+0.0i  # CSGL
      n374 = Variant To Data(error in=w978, type=w983, Variant=w977) -> (data=w974:csg, error out=w975:errorcluster)
      n375 = Complex To Re/Im(x + iy=w974) -> (x=w969:sgl, y=w970:sgl)
      n376 = Bundle(w969, w970) -> (w973:cluster{sgl, sgl})  [unwired: 1 in]
      n377 = Absolute Value(x=w973) -> (abs(x)=w980:cluster{sgl, sgl})
      n378 = Equal To 0?(x=w973) -> (x = 0?=w979:cluster{bool, bool})
      n379 = In Range and Coerce(upper limit=1000000.0, x=w980, lower limit=9.999999747378752e-05 ("upper limit")) -> (In Range?=w972:cluster{bool, bool})  [unwired: 1 out]
      n380 = Or(x=w979, y=w972) -> (x .or. y?=w971:cluster{bool, bool})
      n381 = Unbundle(w971) -> (w965:bool, w964:bool)
      n382 = Select(t=w966, s=w965, f=w967) -> (s? t:f=w968:string)
      n383 = Select(t=w966, s=w964, f=w967) -> (s? t:f=w976:string)
      n384 = Format Value(format string=w968, value (0)=w969) -> (output string=w963:string)  [unwired: 1 in]
      n385 = Format Value(format string=w976, value (0)=w970) -> (output string=w961:string)  [unwired: 1 in]
      n386 = Concatenate Strings(w963, " + " ("string"), w961, " i" ("string")) -> (w960:string)
    }
    frame "Double Complex" {
      w992 = "%#_15e" ("format string")
      w991 = "%#_15f" ("format string")
      w1008 = cdb 0.0+0.0i  # CDBL
      n387 = Variant To Data(error in=w1003, type=w1008, Variant=w1002) -> (data=w999:cdb, error out=w1000:errorcluster)
      n388 = Complex To Re/Im(x + iy=w999) -> (x=w994:dbl, y=w995:dbl)
      n389 = Bundle(w994, w995) -> (w998:cluster{dbl, dbl})  [unwired: 1 in]
      n390 = Absolute Value(x=w998) -> (abs(x)=w1005:cluster{dbl, dbl})
      n391 = Equal To 0?(x=w998) -> (x = 0?=w1004:cluster{bool, bool})
      n392 = In Range and Coerce(upper limit=1000000.0, x=w1005, lower limit=9.999999747378752e-05 ("upper limit")) -> (In Range?=w997:cluster{bool, bool})  [unwired: 1 out]
      n393 = Or(x=w1004, y=w997) -> (x .or. y?=w996:cluster{bool, bool})
      n394 = Unbundle(w996) -> (w990:bool, w989:bool)
      n395 = Select(t=w991, s=w990, f=w992) -> (s? t:f=w993:string)
      n396 = Select(t=w991, s=w989, f=w992) -> (s? t:f=w1001:string)
      n397 = Format Value(format string=w993, value (0)=w994) -> (output string=w988:string)  [unwired: 1 in]
      n398 = Format Value(format string=w1001, value (0)=w995) -> (output string=w986:string)  [unwired: 1 in]
      n399 = Concatenate Strings(w988, " + " ("string"), w986, " i" ("string")) -> (w985:string)
    }
    frame "Extended Complex" {
      w1017 = "%#_18e" ("format string")
      w1016 = "%#_18f" ("format string")
      w1033 = cxt 0.0+0.0i  # CXT
      n400 = Variant To Data(error in=w1028, type=w1033, Variant=w1027) -> (data=w1024:cxt, error out=w1025:errorcluster)
      n401 = Complex To Re/Im(x + iy=w1024) -> (x=w1019:ext, y=w1020:ext)
      n402 = Bundle(w1019, w1020) -> (w1023:cluster{ext, ext})  [unwired: 1 in]
      n403 = Absolute Value(x=w1023) -> (abs(x)=w1030:cluster{ext, ext})
      n404 = Equal To 0?(x=w1023) -> (x = 0?=w1029:cluster{bool, bool})
      n405 = In Range and Coerce(upper limit=1000000.0, x=w1030, lower limit=9.999999747378752e-05 ("upper limit")) -> (In Range?=w1022:cluster{bool, bool})  [unwired: 1 out]
      n406 = Or(x=w1029, y=w1022) -> (x .or. y?=w1021:cluster{bool, bool})
      n407 = Unbundle(w1021) -> (w1015:bool, w1014:bool)
      n408 = Select(t=w1016, s=w1015, f=w1017) -> (s? t:f=w1018:string)
      n409 = Select(t=w1016, s=w1014, f=w1017) -> (s? t:f=w1026:string)
      n410 = Format Value(format string=w1018, value (0)=w1019) -> (output string=w1013:string)  [unwired: 1 in]
      n411 = Format Value(format string=w1026, value (0)=w1020) -> (output string=w1011:string)  [unwired: 1 in]
      n412 = Concatenate Strings(w1013, " + " ("string"), w1011, " i" ("string")) -> (w1010:string)
    }
    frame "Fixed Point" {
      w1055 = ext 0.0  # EXT
      n413 = call <vilib>:"Get Fixed-Point Information.vi"("error in (no error)"=w1043, "variant"=w1041) -> ("error out"=w1042:errorcluster, "FXP representation"=w1044:T6)  [unwired: 6 in, 2 out]
      n414 = Unbundle By Name(w1044) -> ("Word Length"=w1040:u32)
      n415 = Variant To Data(error in=w1042, type=w1055, Variant=w1041) -> (data=w1047:ext, error out=w1045:errorcluster)
      n416 = Absolute Value(x=w1047) -> (abs(x)=w1051:ext)
      n417 = Equal To 0?(x=w1047) -> (x = 0?=w1050:bool)
      n418 = expression code="floor(x*ln(2)/ln(10))"(w1040) -> (w1039:u32)
      n419 = In Range and Coerce(upper limit=1000000.0, x=w1051, lower limit=9.999999747378752e-05 ("upper limit")) -> (In Range?=w1049:bool)  [unwired: 1 out]
      n420 = Or(x=w1049, y=w1050) -> (x .or. y?=w1048:bool)
      n421 = Select(t="f" ("format string"), s=w1048, f="e" ("format string")) -> (s? t:f=w1036:string)
      n422 = Number To Decimal String(number=w1039) -> (decimal integer string=w1037:string)  [unwired: 1 in]
      n423 = Concatenate Strings("%#_" ("format string"), w1037, w1036) -> (w1034:string)
      n424 = Format Value(format string=w1034, value (0)=w1047) -> (output string=w1046:string)  [unwired: 1 in]
    }
    frame "Boolean" {
      n425 = Variant To Data(error in=w1059, type=FALSE, Variant=w1057) -> (data=w1060:bool, error out=w1058:errorcluster)
      n426 = Select(t="True" ("format string"), s=w1060, f="False" ("format string")) -> (s? t:f=w1056:string)
    }
    frame "String" {
      w1066 = "\""
      n427 = Variant To Data(error in=w1069, type="" ("String"), Variant=w1068) -> (data=w1067:string, error out=w1064:errorcluster)
      n428 = Concatenate Strings(w1066, w1067, w1066) -> (w1065:string)
    }
    frame "Path" {
      w1075 = "\""
      n429 = Variant To Data(error in=w1078, type=path "", Variant=w1077) -> (data=w1076:path, error out=w1073:errorcluster)
      n430 = Path To String(path=w1076) -> (string=w1071:string)
      n431 = Concatenate Strings(w1075, w1071, w1075) -> (w1074:string)
    }
    frame "Cluster" {
      n432 = call <vilib>:"Get Cluster Information.vi"("error in (no error)"=w1093, "variant"=w1082) -> ("error out"=w1085:errorcluster, "cluster elements"=w1083:variant[])  [unwired: 8 in]
      n433 = Variant To Data(error in=w1085, type=w1083, Variant=w1082) -> (data=w1081:variant[], error out=w1084:errorcluster)
      n434 = for {
        shift-right: [w1098] -> w1092
        shift-left: w1084 -> [w1099]
        tunnel: w1081 -> [w1097] mode=indexing
        tunnel: [w1096] -> w1088 mode=indexing
        tunnel: w1086 -> [w1095]
        tunnel: w1079 -> [w1094]
        n435 = call "_DRIVER_SHARED_INI_VariantToLegibleString.vi"("Format Options"=w1095, "Preferred Units"=w1094, "error in (no error)"=w1099, "Variant"=w1097) -> ("error out"=w1098:errorcluster, "String"=w1096:string)  [unwired: 4 in, 2 out]
      }
      n436 = call <vilib>:"1D String Array to Delimited String.vi"("delimiter"=";", "string array"=w1088) -> ("delimited string"=w1087:string)  [unwired: 9 in]
      n437 = Concatenate Strings("{", w1087, "}") -> (w1089:string)
    }
    frame "Array" {
      n438 = call <vilib>:"Get Array Information.vi"("error in (no error)"=w1113, "variant"=w1110) -> ("error out"=w1111:errorcluster, "array element data type"=w1108:variant, "number of dimensions"=w1109:i32)  [unwired: 6 in, 1 out]
      n439 = case shown="3" w1109 {
        tunnel: [w1116 w1127 w1144 w1162] -> w1112
        tunnel: [w1114 w1119 w1137 w1155] -> w1104
        tunnel: w1111 -> [w1116 w1126 w1143 w1161]
        tunnel: w1110 -> [_ w1124 w1141 w1159]
        tunnel: w1108 -> [_ w1122 w1140 w1158]
        tunnel: w1101 -> [_ w1118 w1135 w1153]
        tunnel: w1100 -> [_ w1117 w1134 w1152]
        frame 0, Default {
          # "Arrays of greater dimension"
          n440 = Build Array("[Arrays beyond the 3rd dimension not supported]") -> (w1114:string[])
        }
        frame 1 {
          # "1D arrays"
          n441 = Initialize Array(w1122, 0 ("dimension size")) -> (w1121:variant[])
          n442 = Variant To Data(error in=w1126, type=w1121, Variant=w1124) -> (data=w1120:variant[], error out=w1125:errorcluster)
          n443 = for {
            shift-right: [w1132] -> w1127
            shift-left: w1125 -> [w1133]
            tunnel: w1120 -> [w1131] mode=indexing
            tunnel: [w1130] -> w1119 mode=indexing
            tunnel: w1118 -> [w1129]
            tunnel: w1117 -> [w1128]
            n444 = call "_DRIVER_SHARED_INI_VariantToLegibleString.vi"("Format Options"=w1129, "Preferred Units"=w1128, "error in (no error)"=w1133, "Variant"=w1131) -> ("error out"=w1132:errorcluster, "String"=w1130:string)  [unwired: 4 in, 2 out]
          }
        }
        frame 2 {
          w1136 = 0 ("dimension size")
          # "2D arrays"
          n445 = Initialize Array(w1140, w1136, w1136) -> (w1139:variant[][])
          n446 = Variant To Data(error in=w1143, type=w1139, Variant=w1141) -> (data=w1138:variant[][], error out=w1142:errorcluster)
          n447 = for {
            shift-right: [w1150] -> w1144
            shift-left: w1142 -> [w1151]
            tunnel: w1138 -> [w1149] mode=indexing
            tunnel: [w1148] -> w1137 mode=indexing
            tunnel: w1135 -> [w1146]
            tunnel: w1134 -> [w1145]
            n448 = To Variant(anything=w1149) -> (Variant=w1147:variant)
            n449 = call "_DRIVER_SHARED_INI_VariantToLegibleString.vi"("Format Options"=w1146, "Preferred Units"=w1145, "error in (no error)"=w1151, "Variant"=w1147) -> ("error out"=w1150:errorcluster, "String"=w1148:string)  [unwired: 4 in, 2 out]
          }
        }
        frame 3 {
          w1154 = 0 ("dimension size")
          # "3D arrays"
          n450 = Initialize Array(w1158, w1154, w1154, w1154) -> (w1157:variant[][][])
          n451 = Variant To Data(error in=w1161, type=w1157, Variant=w1159) -> (data=w1156:variant[][][], error out=w1160:errorcluster)
          n452 = for {
            shift-right: [w1168] -> w1162
            shift-left: w1160 -> [w1169]
            tunnel: w1156 -> [w1167] mode=indexing
            tunnel: [w1166] -> w1155 mode=indexing
            tunnel: w1153 -> [w1164]
            tunnel: w1152 -> [w1163]
            n453 = To Variant(anything=w1167) -> (Variant=w1165:variant)
            n454 = call "_DRIVER_SHARED_INI_VariantToLegibleString.vi"("Format Options"=w1164, "Preferred Units"=w1163, "error in (no error)"=w1169, "Variant"=w1165) -> ("error out"=w1168:errorcluster, "String"=w1166:string)  [unwired: 4 in, 2 out]
          }
        }
      }
      n455 = call <vilib>:"1D String Array to Delimited String.vi"("delimiter"=";", "string array"=w1104) -> ("delimited string"=w1107:string)  [unwired: 9 in]
      n456 = Concatenate Strings("[", w1107, "]") -> (w1103:string)
    }
    frame "LV Variant" {
      n457 = To Variant(anything=variant) -> (Variant=w1177:variant)
      n458 = Equal?(x=w1177, y=w1172) -> (x = y?=w1176:bool)
      n459 = case shown="False" w1176 {
        tunnel: [w1182 w1189] -> w1175
        tunnel: w1174 -> [w1187 w1189]
        tunnel: [w1181 "<Null>"] -> w1173
        tunnel: w1172 -> [w1186 _]
        tunnel: w1171 -> [w1180 _]
        tunnel: w1170 -> [w1179 _]
        frame False {
          n460 = Variant To Data(error in=w1187, type=variant, Variant=w1186) -> (data=w1183:variant, error out=w1184:errorcluster)
          n461 = call "_DRIVER_SHARED_INI_VariantToLegibleString.vi"("Format Options"=w1180, "Preferred Units"=w1179, "error in (no error)"=w1184, "Variant"=w1183) -> ("error out"=w1182:errorcluster, "String"=w1181:string)  [unwired: 4 in, 2 out]
        }
        frame True {
        }
      }
    }
    frame "Waveform" {
      n462 = Variant To Data(error in=w1203, type=waveform(dbl) {"t0"=timestamp(0 s since 1904-01-01), "dt"=1.0, "Y"=[]} ("Waveform"), Variant=w1201) -> (data=w1198:waveform(dbl), error out=w1200:errorcluster)
      n463 = Unbundle By Name(w1198) -> ("t0"=w1196:timestamp, "dt"=w1195:dbl, "Y"=w1194:dbl[])
      n464 = Bundle By Name(cluster=cluster{"t0":timestamp, "dt":dbl, "y":dbl[]} {"t0"=timestamp(0 s since 1904-01-01), "dt"=1.0, "y"=[]}, "t0"=w1196, "dt"=w1195, "y"=w1194) -> (w1193:cluster{"t0":timestamp, "dt":dbl, "y":dbl[]})
      n465 = To Variant(anything=w1193) -> (Variant=w1192:variant)
      n466 = call "_DRIVER_SHARED_INI_VariantToLegibleString.vi"("Format Options"=w1191, "Preferred Units"=w1190, "error in (no error)"=w1200, "Variant"=w1192) -> ("error out"=w1204:errorcluster, "String"=w1202:string)  [unwired: 4 in, 2 out]
    }
    frame "Timestamp" {
      n467 = Unbundle By Name(w1210) -> ("ISO8601 Timestamps"=w1205:bool)
      n468 = Variant To Data(error in=w1213, type=timestamp(0 s since 1904-01-01), Variant=w1212) -> (data=w1209:timestamp, error out=w1208:errorcluster)
      n469 = case shown="True" w1205 {
        tunnel: w1209 -> [w1225 w1229]
        tunnel: w1208 -> [w1220 w1227]
        tunnel: [w1219 w1227] -> w1207
        tunnel: [w1215 w1226] -> w1206
        frame True {
          # "Crop seconds off timezone and remove '+' if timezone is negative."
          n470 = Format Date/Time String(time format string (%c)="%Y-%m-%dT%H:%M:%S%3u+%z", seconds (now)=w1225) -> (date/time string=w1221:string)  [unwired: 1 in]
          n471 = String Length(string=w1221) -> (length=w1224:i32)
          n472 = Subtract(x=w1224, y=3) -> (x-y=w1222:i32)
          n473 = String Subset(string=w1221, length (rest)=w1222) -> (substring=w1218:string)  [unwired: 1 in]
          n474 = Search and Replace String(input string=w1218, search string="+-", replace string="-" ("replace string (\"\")"), error in=w1220) -> (result string=w1215:string, error out=w1219:errorcluster)  [unwired: 4 in, 2 out]
        }
        frame False {
          n475 = Format Date/Time String(time format string (%c)="", seconds (now)=w1229) -> (date/time string=w1226:string)  [unwired: 1 in]
        }
      }
    }
    frame "Refnum" {
      n476 = call <vilib>:"Get Refnum Information.vi"("error in (no error)"=w1234, "variant"=w1231) -> ("error out"=w1233:errorcluster, "strict type"=w1230:variant, "reference type"=w1232:T7)  [unwired: 6 in, 1 out]
      n477 = case shown="\"Generic\", \"LVObjUnknown\"" w1232 {
        tunnel: [w1238 w1247 w1252 w1262] -> w1236
        tunnel: ["<Unsupported Refnum>" ("Name") w1241 w1249 w1259] -> w1235
        tunnel: w1233 -> [w1238 w1240 w1256 w1265]
        tunnel: w1231 -> [_ w1239 w1255 w1264]
        tunnel: w1230 -> [_ _ _ _]
        frame "NotARefnum", Default {
        }
        frame "Generic", "LVObjUnknown" {
          w1244 = u32 0  # U32
          n478 = Variant To Data(error in=w1240, type=refnum<vi> refnum ("error in (no error)"), Variant=w1239) -> (data=w1245:refnum<vi>, error out=w1247:errorcluster)
          n479 = Type Cast(type=w1244, x=w1245) -> (*(type *) &x=w1243:u32)
          n480 = Number To Hexadecimal String(1:i16 8 ("width (-)"), 2:w1243) -> (0:w1241:string)
        }
        frame "LVObjVI" {
          w1248 = "\"" ("string")
          n481 = control-ref of="This VI"() -> (w1254:refnum<vi>)
          n482 = Variant To Data(error in=w1256, type=w1254, Variant=w1255) -> (data=w1251:refnum<vi>, error out=w1253:errorcluster)
          n483 = property class="VI"(reference=w1251, error in=w1253) -> (error out=w1252:errorcluster, "Name"=w1250:string)  [unwired: 1 out]
          n484 = Concatenate Strings(w1248, w1250, w1248) -> (w1249:string)
        }
        frame "LVObjApp" {
          w1258 = "\"" ("string")
          n485 = control-ref of="This Application"() -> (w1257:refnum<vi>)
          n486 = Variant To Data(error in=w1265, type=w1257, Variant=w1264) -> (data=w1261:refnum<vi>, error out=w1263:errorcluster)
          n487 = property class="App"(reference=w1261, error in=w1263) -> (error out=w1262:errorcluster, "App.Name"=w1260:string)  [unwired: 1 out]
          n488 = Concatenate Strings(w1258, w1260, w1258) -> (w1259:string)
        }
      }
    }
    frame "VI" {
      n489 = control-ref of="This VI"() -> (w1271:refnum<vi>)
      n490 = Variant To Data(error in=w1272, type=w1271, Variant=w1270) -> (data=w1266:refnum<vi>, error out=w1269:errorcluster)
      n491 = property class="VI"(reference=w1266, error in=w1269) -> (error out=w1268:errorcluster, "Name"=w1267:string)  [unwired: 1 out]
    }
  }
  "Var_Value" <- w16
  n492 = Unbundle By Name("Format Options") -> ("Show Names"=w9:bool, "Hide Root Name"=w10:bool)
  n493 = Not(x=w10) -> (.not. x?=w11:bool)
  n494 = And(x=w9, y=w11) -> (x .and. y?=w8:bool)
  n495 = Empty String/Path?(string/path=w15) -> (empty?=w14:bool)
  n496 = Not(x=w14) -> (.not. x?=w12:bool)
  n497 = And(x=w12, y=w8) -> (x .and. y?=w13:bool)
  n498 = case shown="True" w13 {
    tunnel: [w1274 w1279] -> w19
    tunnel: w18 -> [w1274 w1279]
    tunnel: [w1273 w1275] -> w17
    tunnel: w16 -> [w1273 w1278]
    tunnel: w15 -> [_ w1277]
    frame False {
    }
    frame True {
      # "Add variable name to start of string"
      n499 = Concatenate Strings(w1277, "=" ("string"), w1278) -> (w1275:string)
    }
  }
  "String" <- w17
  "error out" <- w19
